vi "Get Channel Data (Old).vi"(8 "error in":errorcluster, 9 "index":i32, 10 "channel name":string, 11 "refnum in":refnum<file>) -> (0 "error out":errorcluster, 1 "data":dbl[](array[numeric]) format="%.2f", 2 "channel name":string, 3 "refnum out":refnum<file>, 4 "unit label":string, 5 "label":string)   [LabVIEW 2017]
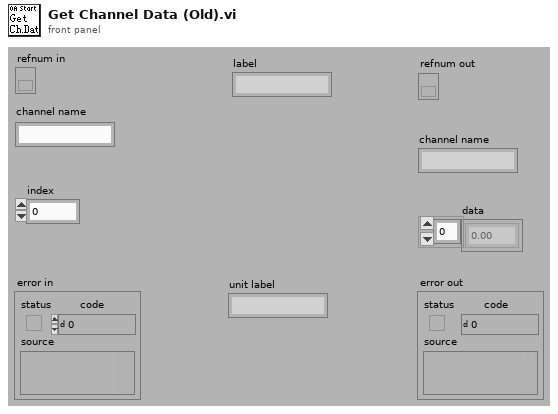
[diagram p1: front panel]
types:
  T1 = cluster{"name":string, "multiplier":sgl, "offset":sgl, "sensor sensitivity (mV/EU)":dbl, "engineering units":enum16{"custom...", "V", "Pa", "g", "m/s^2", "m/s", "m", "in/s^2", "in/s", "in"}}[]
  T2 = cluster{"name":string, "multiplier":sgl, "offset":sgl, "sensor sensitivity (mV/EU)":dbl, "engineering units":enum16{"custom...", "V", "Pa", "g", "m/s^2", "m/s", "m", "in/s^2", "in/s", "in"}}
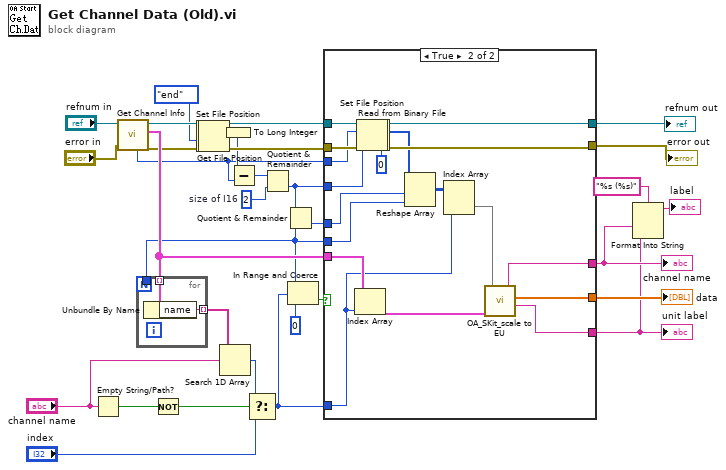
[diagram p0: block diagram]
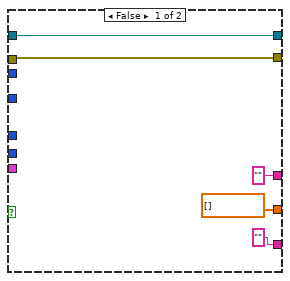
[diagram p2: hidden frame]
diagram:
  w13 = 2  # size of I16
  n1 = Empty String/Path?(string/path="channel name") -> (empty?=w33:bool)
  n2 = call <vilib>:"Get Channel Info.vi"("error in"="error in", "refnum in"="refnum in") -> ("error out"=w20:errorcluster, "channel information"=w25:T1, "dup refnum"=w21:refnum<file>, "data offset"=w10:i32)  [unwired: 4 in, 2 out]
  n3 = for {
    N -> [w35]
    tunnel: w25 -> [w37] mode=indexing
    tunnel: [w36] -> w31 mode=indexing
    tunnel: [w35] -> w8
    n4 = Unbundle By Name(w37) -> ("name"=w36:string)
  }
  n5 = Not(x=w33) -> (.not. x?=w32:bool)
  n6 = Set File Position(refnum=w21, from (0:start)=enum16{"start", "end", "current"}."end" ("pos mode (0:2)"), error in=w20) -> (refnum out=w3:refnum<file>, error out=w2:errorcluster)  [unwired: 1 in]
  n7 = Get File Position(4:w2, 7:w3) -> (0:w23:errorcluster, 2:w1:i64, 3:w22:refnum<file>)
  n8 = Search 1D Array(1D array=w31, element="channel name") -> (index of element=w27:i32)  [unwired: 1 in]
  n9 = To Long Integer(number=w1) -> (32bit integer=w18:i32)
  n10 = Subtract(x=w18, y=w10) -> (x-y=w17:i32)
  n11 = Select(t=w27, s=w32, f="index") -> (s? t:f=w24:i32)
  n12 = Quotient & Remainder(x=w17, y=w13) -> (floor(x/y)=w12:i32)  [unwired: 1 out]
  n13 = Quotient & Remainder(x=w12, y=w8) -> (floor(x/y)=w11:i32)  [unwired: 1 out]
  n14 = In Range and Coerce(upper limit=w8, x=w24, lower limit=0) -> (In Range?=w26:bool)  [unwired: 1 out]
  n15 = case shown="True" w26 {
    tunnel: w25 -> [_ w62]
    tunnel: w24 -> [_ w49]
    tunnel: w22 -> [w39 w59]
    tunnel: w23 -> [w38 w61]
    tunnel: [dbl[] [] ("scaled signal [EU]") w46] -> w16
    tunnel: ["" ("unit label") w45] -> w5
    tunnel: ["" ("name") w58] -> w6
    tunnel: [w38 w53] -> w14
    tunnel: [w39 w57] -> w15
    tunnel: w12 -> [_ w55]
    tunnel: w11 -> [_ w54]
    tunnel: w10 -> [_ w52]
    tunnel: w8 -> [_ w48]
    frame False {
    }
    frame True {
      n16 = Index Array(array=w62, index=w49) -> (element=w60:T2)
      n17 = Set File Position(offset (in bytes) (0)=w52, refnum=w59, error in=w61) -> (refnum out=w44:refnum<file>, error out=w43:errorcluster)  [unwired: 1 in]
      n18 = Read from Binary File(5:i16 0, 8:w43, 10:w55, 11:w44) -> (0:w53:errorcluster, 2:w51:i16[], 3:w57:refnum<file>)  [unwired: 2 in, 1 out]
      n19 = Reshape Array(w51, w54, w48) -> (w50:i16[][])
      n20 = Index Array(array=w50, index (col)=w49) -> (element=w47:i16[])  [unwired: 1 in]
      n21 = call <vilib>:"OA_SKit_scale to EU.vi"("channel information"=w60, "measured data"=w47) -> ("unit lable"=w45:string, "scaled data [EU]"=w46:dbl[], "channel name"=w58:string)  [unwired: 3 in]
    }
  }
  "data" <- w16
  "unit label" <- w5
  "channel name" <- w6
  "refnum out" <- w15
  "error out" <- w14
  n22 = Format Into String(format string="%s (%s)" ("Format String"), w6, w5) -> (resulting string=→"label":string)  [unwired: 2 in, 1 out]
